vi "user initialization.vi"(8 "error in":errorcluster, 10 "configuration in":refnum<class "control module configuration.lvclass">, 11 "fixed channel runtime in":refnum<class "ScaleAndLimitModule runtime.lvclass">) -> (0 "error out":errorcluster, 3 "fixed channel runtime out":refnum<class "ScaleAndLimitModule runtime.lvclass">)   [LabVIEW 2017, in "ScaleAndLimitModule runtime.lvclass"]
uses:
  ScaleAndLimitModule runtime.lvclass
  <vilib>/NI/DCAF/Tag Editor Core/control module/configuration/control module configuration.lvclass
  <vilib>/userdefined/High Color/nirio_resource_hc.ctl
  <vilib>/NI/DCAF/addons/InstructionFrameworkSupport/FPGA_FGV_action.ctl
  configuration/ScaleAndLimitModule configuration.lvclass
  C:/Program Files (x86)/National Instruments/LabVIEW 2017/vi.lib/NI/DCAF/Tag Editor Core/control module/configuration/control module configuration.lvclass
  configuration/ScaleAndLimitModule configuration.lvclass/ScaleAndLimitModule configuration.ctl
  ScaleAndLimitModule runtime.lvclass/ScaleAndLimitModule runtime.ctl
  configuration/Read ScaleAndLimitConfig.vi
  <instrlib>/_niInstr/FIFO Register Bus/v1/Host/niInstr FIFO Register Bus v1 Host.lvclass
  C:/Program Files (x86)/National Instruments/LabVIEW 2017/instr.lib/_niInstr/Instruction Framework/v1/Host/Instruction Target/niInstr Instruction Target v1 Host.lvclass
  <vilib>/NI/DCAF/Tag Editor Core/control module/runtime/control module runtime.lvclass
  <vilib>/NI/PowerElectronicsControl/ScaleAndLimit/Interface/ScaleAndLimitInterface.lvlib
  <instrlib>/_niInstr/Instruction Framework/v1/Host/Subsystem Map/niInstr Subsystem Map v1 Host.lvclass
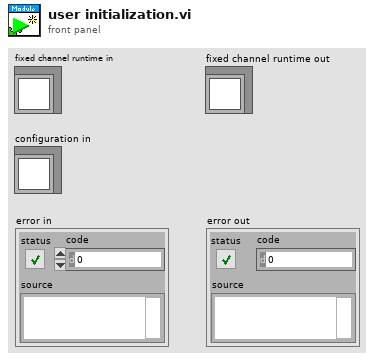
[diagram p1: front panel]
types:
  T1 = typedef "FPGA_FGV_action.ctl" = enum16{"get FPGA", "set FPGA", "Close"}
  T2 = typedef "nirio_resource_hc.ctl" = tag
  T3 = typedef "ScaleAndLimitInterface.lvlib/Configuration.ctl" = cluster{"Name":string, "M":dbl, "B":i16, "HighLimit":dbl, "LowLimit":dbl, "LimitsEnabled":bool}
  T4 = typedef "ScaleAndLimitInterface.lvlib/Interface.ctl" = cluster{"instruction target":refnum<class "niInstr Instruction Target v1 Host.lvclass">, "ScalingAndLimitsContext":refnum<class "niInstr Instruction Framework Context v1 Host.lvclass">, "Configuration":T3[]}
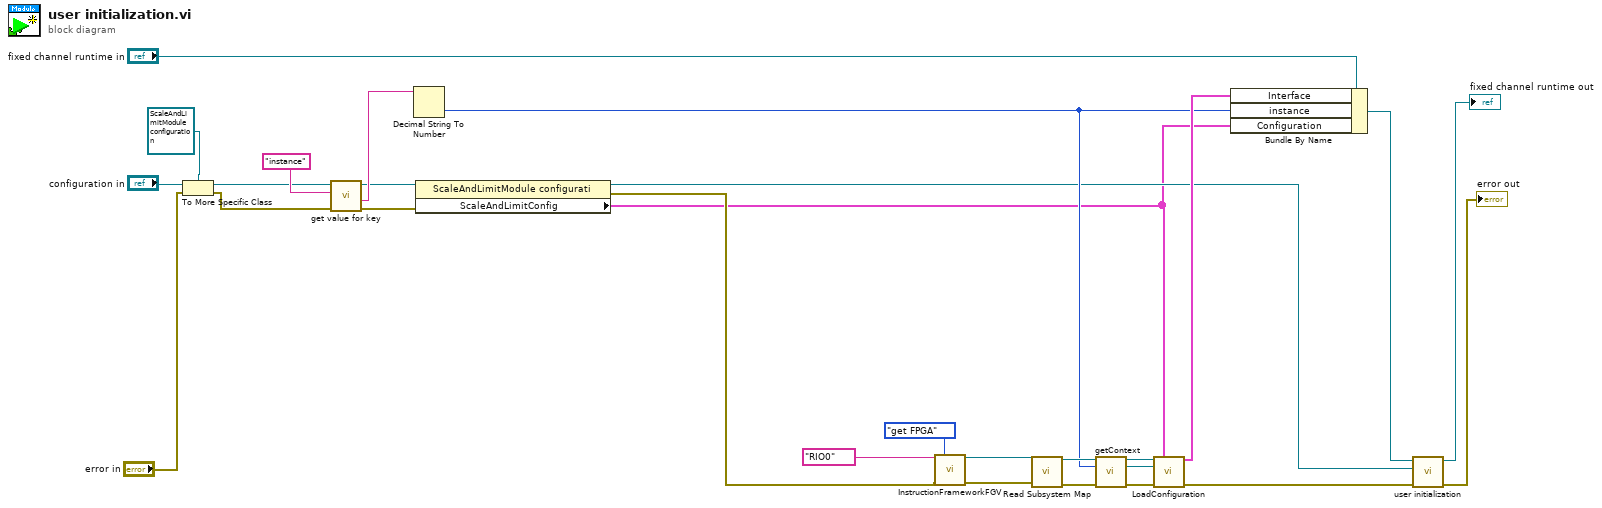
[diagram p0: block diagram]
diagram:
  n1 = To More Specific Class(target class=refnum<class "ScaleAndLimitModule configuration.lvclass"> refnum ("ScaleAndLimitModule configuration"), reference="configuration in", error in="error in") -> (specific class reference=w5:refnum<class "ScaleAndLimitModule configuration.lvclass">, error out=w3:errorcluster)
  n2 = call-dynamic "get value for key.vi"("error in"=w3, "key"="instance", "fixed channel configuration in"=w5) -> ("error out"=w9:errorcluster, "value"=w16:string, "fixed channel configuration out"=w10:refnum<class "ScaleAndLimitModule configuration.lvclass">)  [unwired: 6 in]
  n3 = Decimal String To Number(string=w16) -> (number=w15:i32)  [unwired: 2 in, 1 out]
  n4 = property class="ScaleAndLimitModule configurati"(reference=w10, error in=w9) -> (reference out=w8:refnum<class "ScaleAndLimitModule configuration.lvclass">, error out=w7:errorcluster, "ScaleAndLimitConfig"=w1:T3[])
  n5 = call <vilib>:"InstructionFrameworkFGV.vi"("RIO resource"=T2 "RIO0", "Action"=FPGA_FGV_action."get FPGA", "error in"=w7) -> ("session out"=w11:refnum<class "niInstr FIFO Register Bus v1 Host.lvclass">, "error out"=w12:errorcluster)  [unwired: 10 in, 1 out]
  n6 = call <instrlib>:"Read Subsystem Map.vi"("instruction target in"=w11, "error in"=w12) -> ("instruction target out"=w25:refnum<class "niInstr FIFO Register Bus v1 Host.lvclass">, "error out"=w19:errorcluster)  [unwired: 11 in, 1 out]
  n7 = call <vilib>:"getContext.vi"("session in"=w25, "instance"=w15, "error in"=w19) -> ("session out"=w24:refnum<class "niInstr FIFO Register Bus v1 Host.lvclass">, "ScalingAndLimitsContext"=w23:refnum<class "niInstr Instruction Framework Context v1 Host.lvclass">, "error out"=w20:errorcluster)  [unwired: 10 in]
  n8 = call <vilib>:"LoadConfiguration.vi"("instruction target in"=w24, "Configuration"=w1, "ScalingAndLimitsContext"=w23, "error in (no error)"=w20) -> ("Interface"=w21:T4, "error out"=w18:errorcluster)  [unwired: 10 in]
  n9 = Bundle By Name(cluster="fixed channel runtime in", "Interface"=w21, "instance"=w15, "Configuration"=w1) -> (w26:refnum<class "ScaleAndLimitModule runtime.lvclass">)
  n10 = call-parent "user initialization.vi"("error in"=w18, "configuration in"=w8, "fixed channel runtime in"=w26) -> ("error out"=→"error out":errorcluster, "fixed channel runtime out"=→"fixed channel runtime out":refnum<class "ScaleAndLimitModule runtime.lvclass">)  [unwired: 7 in]
